vi "DriveForTime.vi"() -> ()   [LabVIEW 2017]
panel:
  in  "Time":u32
  in  "Speed":dbl
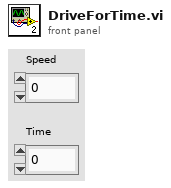
[diagram p1: front panel]
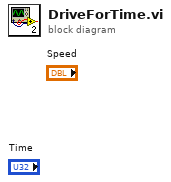
[diagram p0: block diagram]
diagram:
